vi "Ctor.vi"(8 "error in (no error)":errorcluster, 11 "Resource in":refnum<class "Resource.lvclass">) -> (0 "error out":errorcluster, 3 "Resource out":refnum<class "Resource.lvclass">)   [LabVIEW 2020, in "PicoG-Core.lvlib" / "Resource.lvclass"]
uses:
  Resource.lvclass
  Resource.lvclass/Resource.ctl
  <vilib>/IlluminatedG/lv-stream/stream/Stream.lvclass
  Ref Data.ctl
  <vilib>/IlluminatedG/lv-stream/Connection/Connection.lvclass
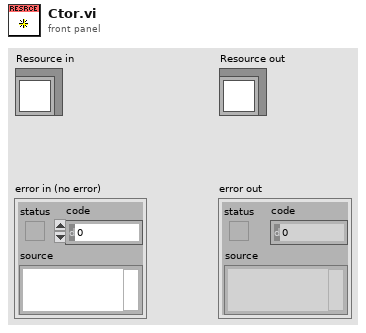
[diagram p1: front panel]
types:
  T1 = typedef "PicoG-Core.lvlib/Resource.lvclass/Ref Data.ctl" = cluster{"Config":map{string, string}, "Stream":refnum<class "Stream.lvclass">}
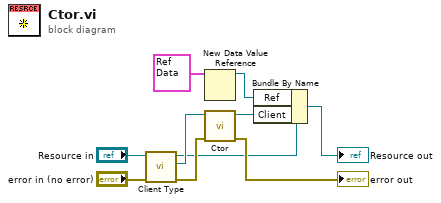
[diagram p0: block diagram]
diagram:
  n1 = call-dynamic "Client Type.vi"("error in (no error)"="error in (no error)", "Resource in"="Resource in") -> ("error out"=w4:errorcluster, "Client"=w5:refnum<class "Connection.lvclass">, "Resource out"=w3:refnum<class "Resource.lvclass">)  [unwired: 7 in]
  n2 = New Data Value Reference(data value=T1 {"Config"={}, "Stream"=refnum} ("Ref Data")) -> (data value reference=w9:refnum<data-value>)  [unwired: 1 in, 1 out]
  n3 = call-dynamic "Ctor.vi"("error in (no error)"=w4, "Connection in"=w5) -> ("error out"=→"error out":errorcluster, "Connection out"=w1:refnum<class "Connection.lvclass">)  [unwired: 8 in]
  n4 = Bundle By Name(cluster=w3, "Ref"=w9, "Client"=w1) -> (→"Resource out":refnum<class "Resource.lvclass">)
